vi "Stub_Custom ErrorClass.vi"(8 "error in":errorcluster, 11 "Class":refnum<class>) -> (0 "error out":errorcluster)   [LabVIEW 2020]
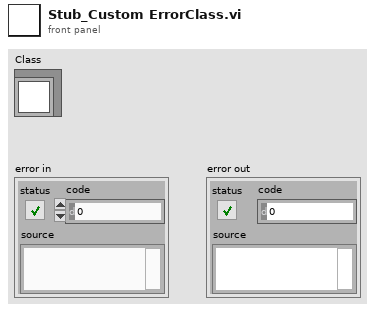
[diagram p1: front panel]
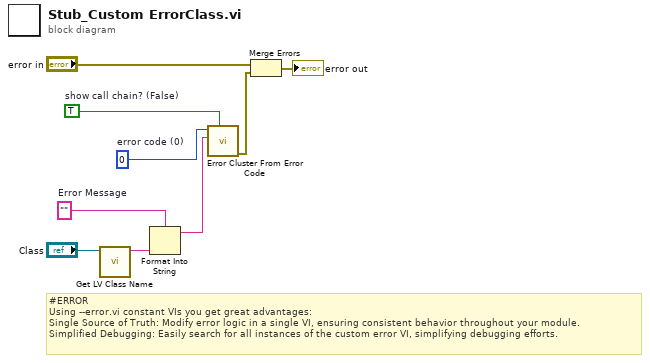
[diagram p0: block diagram]
diagram:
  w5 = 0  # error code (0)
  w3 = ""  # Error Message
  w6 = TRUE  # show call chain? (False)
  # "#ERROR\nUsing --error.vi constant VIs you get great advantages:\nSingle Source of Truth: Modify error logic in a single VI, ensuring consistent behavior throughout your module.\nSimplified Debugging: Easily search for all instances of the custom error VI, simplifying debugging efforts."
  n1 = call <vilib>:"Get LV Class Name.vi"("object"="Class") -> ("class name"=w1:string)  [unwired: 9 in, 1 out]
  n2 = Format Into String(format string=w3, w1) -> (resulting string=w4:string)  [unwired: 2 in, 1 out]
  n3 = call <vilib>:"Error Cluster From Error Code.vi"("show call chain? (False)"=w6, "error message (\"\")"=w4, "error code (0)"=w5) -> ("error out"=w9:errorcluster)  [unwired: 6 in]
  n4 = Merge Errors("error in", w9) -> (→"error out":errorcluster)
